vi "List-Remove Current Item.vi"(11 "List in":refnum<vi>) -> (3 "List Out":refnum<vi>)   [LabVIEW 2024]
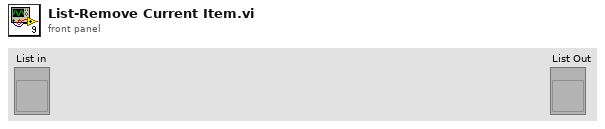
[diagram p1: front panel]
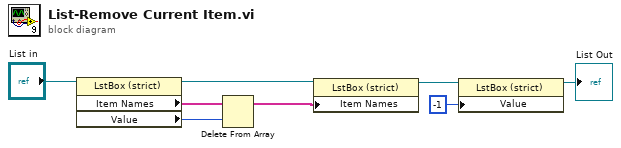
[diagram p0: block diagram]
diagram:
  n1 = property class="LstBox (strict)"(reference="List in") -> (reference out=w5:refnum<vi>, "Item Names"=w7:string[], "Value"=w6:i32)  [unwired: 1 in, 1 out]
  n2 = Delete From Array(array=w7, index=w6) -> (array with subset deleted=w4:string[])  [unwired: 1 in, 1 out]
  n3 = property class="LstBox (strict)"(reference=w5, "Item Names"=w4) -> (reference out=w3:refnum<vi>)  [unwired: 1 in, 1 out]
  n4 = property class="LstBox (strict)"(reference=w3, "Value"=-1) -> (reference out=→"List Out":refnum<vi>)  [unwired: 1 in, 1 out]
